vi "LIA_FPGA.vi"() -> (0 "R":fxp<+,1,1>, 1 "K Constant":fxp<+/-,32,16>, 2 "Nominal Freq":fxp<+/-,64,32>, 3 "phase (pi)":fxp<+/-,16,2>)   [LabVIEW 2012]
uses:
  <vilib>/rvi/DataTransferAndStorage/Container/Common/niFpgaContainerMetaDataKey.ctl
  <vilib>/rvi/DataTransferAndStorage/Container/Common/niFpgaContainerState.ctl
  <vilib>/rvi/DataTransferAndStorage/Container/Common/niFpgaDataTypeControl.ctl
  <vilib>/rvi/DataTransferAndStorage/Container/Common/niFpgaContainerImplementationControl.ctl
  <vilib>/rvi/DataTransferAndStorage/Container/Common/niFpgaContainerArbitrationOptionsControl.ctl
  <vilib>/rvi/DataTransferAndStorage/Container/Common/niFpgaTransferTypeControl.ctl
  <vilib>/rvi/DataTransferAndStorage/Container/Common/niFpgaContainerInitializationParameters.ctl
  <vilib>/rvi/Memory/Memory_Types/niFpgaMemoryInterfaceConfiguration.ctl
  <vilib>/rvi/FIFO/Fifo_Types/niFpgaFifoControlLogicControl.ctl
  <vilib>/Platform/TimedLoop/XDataNode/timing_clust.ctl
  <vilib>/Platform/TimedLoop/XDataNode/nitl_modes.ctl
  <vilib>/Platform/TimedLoop/XDataNode/wakeup.ctl
  <vilib>/rvi/FXPMathLib/FxpRectToPolar/subVIs/nifxpmath_RectToPolar_SimConfig.ctl
  <vilib>/rvi/FXPMathLib/FxpDiv/subVIs/nifxpmath_Div_SimConfig.ctl
  <vilib>/rvi/DataTransferAndStorage/Container/Common/niFpgaContainerGetUniqueNameForEmu.vi
  <vilib>/rvi/DataTransferAndStorage/Container/Common/niFpgaContainerSetEmuInfo.vi
  <vilib>/rvi/eio/common/nirviEmuReportErrorAndStop.vi
  <vilib>/rvi/FXPMathLib/FxpRectToPolar/simVIs/DllFxpRectToPolarTemp_sub.vi
  <vilib>/rvi/FXPMathLib/FxpDiv/simVIs/DllFxpDivTemp_sub.vi
  <vilib>/rvi/eio/common/nirviEmuTemplateMethod_errors.vi
  <vilib>/rvi/Emulation/niFpgaSctlEmulationGetInTimedLoop.vi
  <vilib>/rvi/FIFO/Fifo_Resource/nirvififoEmulationSetSize.vi
  <vilib>/rvi/errors/niFpgaSetErrorForExecOnDevCompSimple.vi
  <vilib>/rvi/Emulation/niFpgaSctlEmulationFifoFullMgr.vi
  <vilib>/rvi/Emulation/niFpgaSctlEmulationResourceMgr.vi
  <vilib>/rvi/Emulation/niFpgaSctlEmulationRegisterWithScheduler.vi
  <vilib>/rvi/Emulation/niFpgaSctlEmulationScheduler.vi
  <vilib>/rvi/LocalResourceManager/LocalResourceManager.xnode
  <vilib>/Platform/TimedLoop/XDataNode/XDataNode.xnode
  <vilib>/rvi/FXPMathLib/FxpRectToPolar/XNode/nifxpmath_RectToPolar.xnode
  <vilib>/rvi/FXPMathLib/FxpDiv/XNode/nifxpmath_Div.xnode
  <vilib>/rvi/FXPMathLib/FxpMul/XNode/nifxpmath_Multiplier.xnode
  <vilib>/rvi/FXPMathLib/FxpInterpret/XNode/nifxpmath_Interpret.xnode
  <vilib>/eio/EIONode/EIONode.xnode
  <vilib>/rvi/DataTransferAndStorage/Container/XNode/niFpgaContainer.xnode
  <vilib>/rvi/FIFO/Fifo_Resource/nirvififoEmulationWrite.vi
  <vilib>/rvi/FIFO/Fifo_Resource/nirvififoEmulationRead.vi
  <vilib>/Platform/TimedLoop/XDataNode/XDNodeRunTimeDep.lvlib
  <vilib>/rvi/FXPMathLib/sim/FxpSim.dll
panel:
  out "Degree":fxp<+,1,1>
  in  "stop 2":bool
  in  "Filter Constant":i64
  in  "Period":u16=1000
  out "ticks":u16
  out "ref":i16 format="%.0x"
  out "sig":i16 format="%.0x"
  out "channelQ":i64
  out "channelI":i64
  out "f":fxp<+/-,32,0> format="%.32g"
  in  "start":bool
  in  "dec2":i16=1
  in  "K":fxp<+,16,0>=0.001007080078125
  in  "nominal freq":fxp<+,16,0>=0.010009765625
  in  "dec1":i16=1
  in  "stages":i8=1
  in  "stop":bool
  in  "decimation":i16=1024
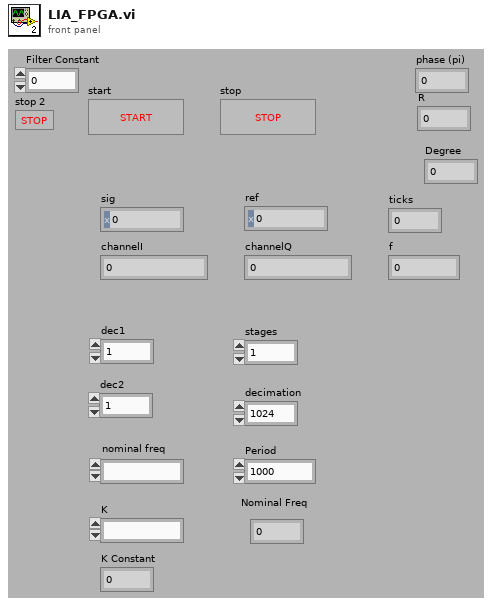
[diagram p1: front panel]
types:
  T1 = typedef "XDNodeRunTimeDep.lvlib/timing_clust.ctl" = cluster{"Expected End [f-1]":u64, "Actual End [f-1]":u64, "Finished Late? [f-1]":bool, "Expected End [i-1]":u64, "Actual End [i-1]":u64, "Finished Late? [i-1]":bool, "Expected Start [i]":u64, "Actual Start [i]":u64, "Expected Start [f]":u64, "Actual Start [f]":u64, "Source Name":string, "Structure Name":string, "Period":i64, "Deadline":i64, "Offset":i64, "Start":i64, "Priority":i32, "Timeout":i32, "Mode":T2, "Wakeup Reason":T3, "Error":errorcluster, "Source Type":string, "Secondary Source Type":string, "Global End Time":u64, "Global Start Time":u64, "Frame Duration":u64, "Iteration Duration":u64, "Assigned CPU":i32, "I/O Scan Engine Mode":u32}
  T2 = typedef "XDNodeRunTimeDep.lvlib/nitl_modes.ctl" = enum32{"No Change", "Process missed periods, maintain original phase", "Discard missed periods, maintain original phase", "Process missed periods, ignore original phase", "Discard missed periods, ignore original phase"}
  T3 = typedef "XDNodeRunTimeDep.lvlib/wakeup.ctl" = enum32{"Normal", "Aborted", "Asynchronous wakeup", "Timing source error", "Timed loop error", "Timeout"}
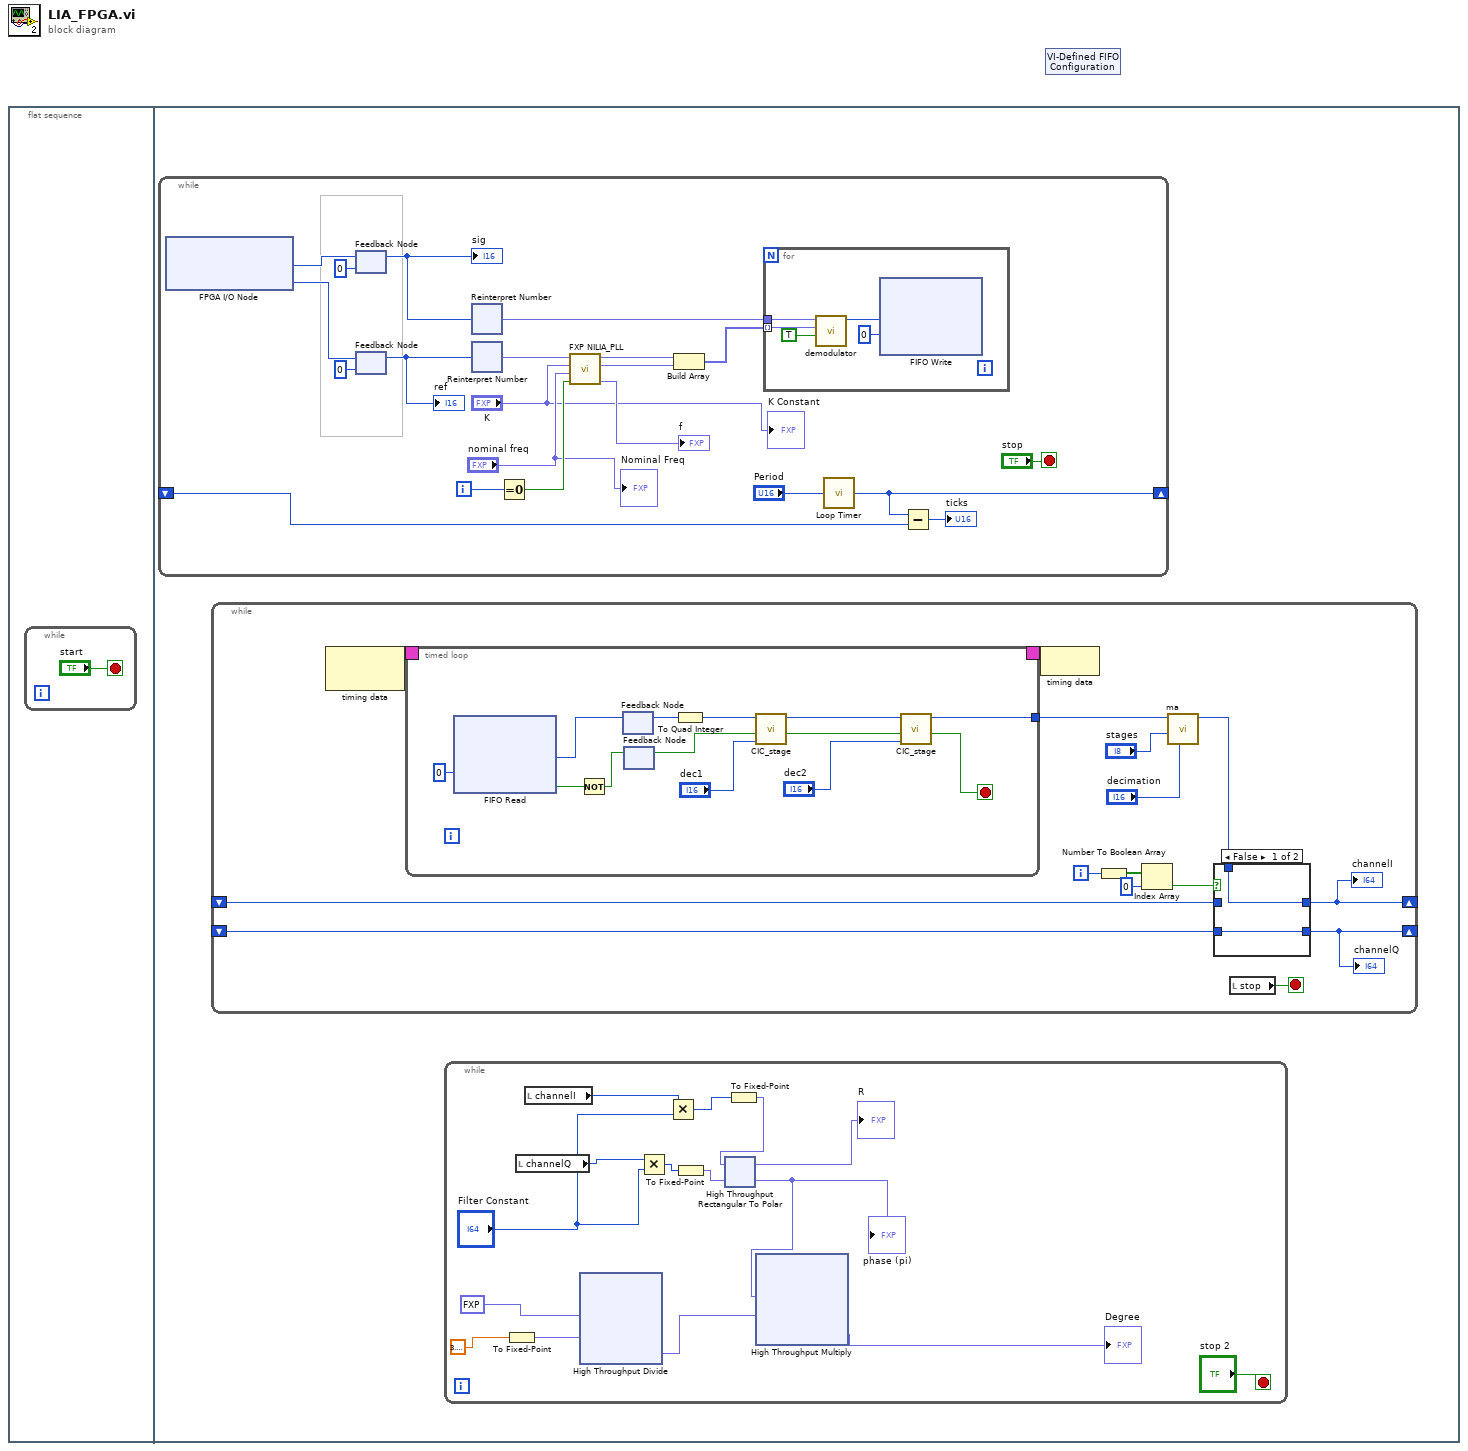
[diagram p0: block diagram]
diagram:
  n1 = flat-sequence {
    frame #0 {
      n2 = while {
        stop <- "start" stop-if-true
      }
    }
    frame #1 {
      n3 = while {
        shift-right: [w98] -> _
        shift-left: _ -> [w97]
        i -> [w101]
        stop <- "stop" stop-if-true
        n4 = xnode "FPGA I/O Node"() -> ("Connector0/AI6"=w91:i16, "Connector0/AI7"=w88:i16)  [unwired: 2 in, 2 out]
        n5 = feedback #1(i16 0 ("y")) -> (w90:i16)
        "sig" <- w90
        n6 = feedback-in #1(w91) -> ()
        n7 = feedback #2(i16 0 ("z [I32.1]")) -> (w89:i16)
        "ref" <- w89
        n8 = feedback-in #2(w88) -> ()
        n9 = xnode "Reinterpret Number"("x"=w90) -> ("y"=w94:fxp<+/-,16,1>)
        n10 = xnode "Reinterpret Number"("x"=w89) -> ("y"=w87:fxp<+/-,16,1>)
        n11 = Equal To 0?(x=w101) -> (x = 0?=w83:bool)
        n12 = call "FXP NILIA_PLL.vi"("reset?"=w83, "norminal freq [U16.0]"="nominal freq", "alpha [U16.0]"="K", "x[I16.1]"=w87) -> ("f"=→"f":fxp<+/-,32,0>, "sin(z)"=w85:fxp<+/-,16,2>, "cos(z)"=w84:fxp<+/-,16,2>)  [unwired: 4 in, 1 out]
        n13 = Build Array(w84, w85) -> (w95:fxp<+/-,16,2>[])
        n14 = for {
          tunnel: w94 -> [w104]
          tunnel: w95 -> [w102] mode=indexing
          n15 = call "demodulator.vi"("New Data"=TRUE, "ref"=w102, "signal"=w104) -> ("x*y"=w105:i32)  [unwired: 8 out]
          n16 = xnode ("FIFO Write")("Element"=w105, "Timeout"=0) -> ()  [unwired: 1 in, 2 out]
        }
        n17 = call "Loop Timer"("Count(Ticks)"="Period") -> ("Tick Count(Ticks)"=w98:u16)
        n18 = Subtract(x=w98, y=w97) -> (x-y=→"ticks":u16)
        "Nominal Freq" <- "nominal freq"
        "K Constant" <- "K"
      }
      n19 = while {
        shift-right: [w108] -> _
        shift-left: _ -> [w110]
        shift-right: [w107] -> _
        shift-left: _ -> [w109]
        i -> [w115]
        stop <- w117 stop-if-true
        n20 = node-c288() -> (w121:T1)  [unwired: 1 out]
        n21 = timed-loop {
          timing: w121 -> [_]
          timing-out: [_] -> w120
          tunnel: [w129] -> w116
          stop <- w128 stop-if-true
          n22 = xnode ("FIFO Read")("Timeout"=0) -> ("Element"=w136:i32, "Timed Out?"=w135:bool)  [unwired: 1 in, 1 out]
          n23 = Not(x=w135) -> (.not. x?=w134:bool)
          n24 = feedback-in #3(w136) -> ()
          n25 = feedback #3() -> (w138:i32)  [unwired: 1 out]
          n26 = feedback-in #4(w134) -> ()
          n27 = feedback #4() -> (w132:bool)  [unwired: 1 out]
          n28 = To Quad Integer(1:w138) -> (0:w133:i64)
          n29 = call "CIC_stage.vi"("decimate factor"="dec1", "New Data"=w132, "input"=w133) -> ("Data Ready"=w130:bool, "output"=w131:i64)  [unwired: 7 out]
          n30 = call "CIC_stage.vi"("decimate factor"="dec2", "New Data"=w130, "input"=w131) -> ("Data Ready"=w128:bool, "output"=w129:i64)  [unwired: 7 out]
        }
        n31 = node-c288(w120) -> ()
        n32 = Number To Boolean Array(number=w115) -> (Boolean array=w114:bool[])
        n33 = Index Array "Index Array"(array=w114, index=0) -> (element=w112:bool)
        n34 = call "ma.vi"("decimate"="decimation", "stages"="stages", "input"=w116) -> ("output"=w111:i64)  [unwired: 8 out]
        n35 = case shown="False" w112 {
          tunnel: w111 -> [w123 w125]
          tunnel: [w123 w124] -> w108
          tunnel: [w122 w125] -> w107
          tunnel: w110 -> [_ w124]
          tunnel: w109 -> [w122 _]
          frame False {
          }
          frame True {
          }
        }
        "channelI" <- w108
        "channelQ" <- w107
        n36 = local read "stop"() -> (w117:bool)
      }
      n37 = while {
        stop <- "stop 2" stop-if-true
        n38 = To Fixed-Point(number=sgl 3.1415927) -> (fixed-point=w3:fxp<+/-,64,64>)  [unwired: 1 in]
        n39 = local read "channelQ"() -> (w15:i64)
        n40 = local read "channelI"() -> (w16:i64)
        n41 = xnode "High Throughput Divide"("x"=fxp<+,6,8> 180.0, "y"=w3) -> ("x/y"=w5:fxp<+/-,9,9>)
        n42 = Multiply(x=w15, y="Filter Constant") -> (x*y=w11:i64)
        n43 = Multiply(x=w16, y="Filter Constant") -> (x*y=w13:i64)
        n44 = To Fixed-Point(number=w11) -> (fixed-point=w10:fxp<+/-,64,64>)  [unwired: 1 in]
        n45 = To Fixed-Point(number=w13) -> (fixed-point=w12:fxp<+/-,64,64>)  [unwired: 1 in]
        n46 = xnode "High Throughput Rectangular To Polar"("x"=w12, "y"=w10) -> ("magnitude"=→"R":fxp<+,64,64>, "phase (pi)"=w6:fxp<+/-,16,2>)
        "phase (pi)" <- w6
        n47 = xnode "High Throughput Multiply"("x"=w6, "y"=w5) -> ("x*y"=→"Degree":fxp<+/-,25,11>)
      }
    }
  }
  n48 = xnode "VI-Defined FIFO Configuration"() -> ()  [unwired: 1 out]
